vi "ADC_Monitor.vi"(0 "GPIB Address":T1=8, 5 "Chunk Size":i32=1000, 9 "Sample Rate (Hz)":dbl, 11 "error in (no error)":errorcluster, 12 "Local Client?":bool, 13 "Current Block No":i32) -> (6 "Barchart":cluster{i32, i32}(slide)={1, 0} scale=0.0..1048576.0, 15 "error out":errorcluster)   [LabVIEW 2010]
doc: "This VI starts a buffered analog input operation. This VI sets the scan rate and trigger conditions and then starts an acquisition.\n\nAI Start first checks to see if the input cluster error in indicates that an error has already occurred. If so, this VI does not start an acquisition, but passes the error information unmodified through error out. \n\nOtherwise, this VI calls several lower-level analog input VIs to start the buffered analog input acquisition. AI Start calls Analog Input Clock Config for the specified taskID to configure the acquisition to use the specified scan clock source (internal by default) and the specified scan rate.\n\nAI Start then calls Analog Input Trigger Config to set a trigger according to trigger type. If trigger type is 0, then it clears the trigger; otherwise it sets the specified type of trigger.\n\nFinally, AI Start calls Analog Input Control to start the acquisition, using total scans, pretrigger scans, and number of buffers to acquire to determine how much data to acquire.\n\nInput Values:\n\n(u32) taskID in: identifies the group and I/O operation.\n\n(i32) number of scans to aquire: the total number of scans to acquire before the acquisition is complete. The default input -1which tells LabVIEW to acquire exactly one buffer of data. The buffer size is specified when AI Config is called. The number of total scans includes any pretrigger scans requested. If you set number of scans to acquire to 0, LabVIEW acquires data indefinitely into the first (or only) buffer until you clear the acquisition with AI Clear. In this case, the VI ignores the pretrigger scans input.\n\n(sgl) scan rate: the number of scans per second to acquire. The default input is 1,000 scans/sec. Refer to the description of the Analog Input Clock Config VI for more options with alternate clock sources.\n\n(i32) number of buffers to acquire: needs to be changed only when you allocate more than one buffer with AI Config or Analog Input Buffer Config for multi-buffered acquisition (see Chapter 1 for a description of different types of I/O operation). If number of buffers to acquire is 0, LabVIEW acquires buffers of data indefinitely. Otherwise, LabVIEW acquires only the specified number of buffers. The default input is 1.\n\n(u16) scan clock source:\n 0: Do not change the clock source setting (default input). \n 1: Internal (default setting). \n 2: I/O connector. \n 3: RTSI connection. \n\n(u16) trigger type: \n 0: Do not change the trigger type setting (default input). \n 1: Analog trigger (default setting). \n 2: Digital trigger A. \n 3: Digital trigger A & B. \n 4: Scan clock gating. \n\n(i32) pretrigger scans: the number of scans to save in the buffer before the trigger. The default input is 0, which tells LabVIEW to acquire all data after the trigger.\n\n(u16) edge or slope:\n 0: Do not change the default setting (default input). \n 1: Rising edge for digital trigger or\n rising slope for analog trigger. \n 2: Falling edge for digital trigger or\n falling slope for analog trigger. \n\n(cluster) analog chan and level: a cluster of the following parameters that are used only when the trigger type is analog:\n\n (string) analog chan: specifies the analog channel\n that is the source of the trigger. Uses the same\n syntax described in the Analog Input Group Config VI,\n with the following exceptions. \n a) An empty string tells LabVIEW not to change \n the trigger source setting (default input).\n b) EXTx denotes an external analog input \n trigger, where x is the channel number.\n Currently, x must be 0. You can substitute\n the string EXTERNAL for EXT.\n \n (sgl) level: the scaled data value the analog source\n must cross for a trigger to occur. You must also\n specify whether level must be crossed on a rising \n or falling slope with the edge or slope input.\n The default input for level is 0.0.\n\n(cluster) additional trig params: a cluster of the following parameters: \n \n (sgl) hysteresis is expressed in scaled data values.\n The default input and setting are 0.0 V. \n \n (u16) coupling:\n 0: Do not change (default input). \n 1: DC. \n 2: AC. \n \n (sgl) delay: expressed in seconds.\n The default input and setting are 0.0 sec (no delay). \n \n (i32) skip count: the number of triggers to\n ignore before triggering the acquisition.\n The default input is -1, use the current default \n setting. The default setting is 0, don't skip \n any triggers. \n \n (sgl) time limit: time limit for software \n triggering. The default input is -1.0, use \n default setting. The default setting is 1.0Êsec. \n\n(cluster) error in: a cluster describing any error conditions prior to this VI's execution. The default input of this cluster is no error. If an error has already occurred, this VI does not start the acquisition, it just passes the values of taskID in and error in to taskID out and error out. The error in cluster contains the following parameters: \n\n (bool) status: TRUE if an error has occurred.\n If status is TRUE, this VI does not start the\n acquisition.\n\n (i32) code: the error code associated with an error.\n A value of 0 means no error, a negative value is an error,\n and a positive value is a warning.\n\n (string) source: an indication of where an \n error occurred, usually the name of the VI.\n\nOutput Values:\n\n(u32) taskID out: the same as taskID in; identifies the group and I/O operation.\n\n(sgl) actual scan rate: may differ slightly from the requested scan rate, depending on the hardware capabilities.\n\n(cluster) actual trigger params: may differ slightly from the requested trigger inputs, depending on the hardware capabilities. It contains the following parameters:\n \n (sgl) actual level: the analog trigger level used.\n \n (sgl) actual hysteresis: the hysteresis used. \n \n (sgl) actual delay: the trigger delay used. \n\n(cluster) error out: a cluster containing error information. If error in indicated an error, error out contains the same error information. Otherwise, it describes the error status of this VI. Use the General Error Handler utility VI to check the error at the end of your diagram. The error out cluster contains the following parameters: \n\n (bool) status: TRUE if an error has occurred.\n\n (i32) code: the error code associated with an error.\n A value of 0 means no error, a negative value is an error,\n and a positive value is a warning.\n\n (string) source: an indication of where an \n error occurred, usually the name of the VI."
uses:
  ADC_GPIB_address.ctl
panel:
  out "Unread samples":i32
  in  "stop":bool
  out "message":string
  # "Read marker"
  # "Write marker"
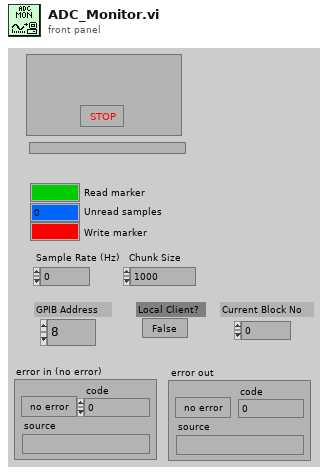
[diagram p1: front panel]
types:
  T1 = typedef "ADC_GPIB_address.ctl" = u8
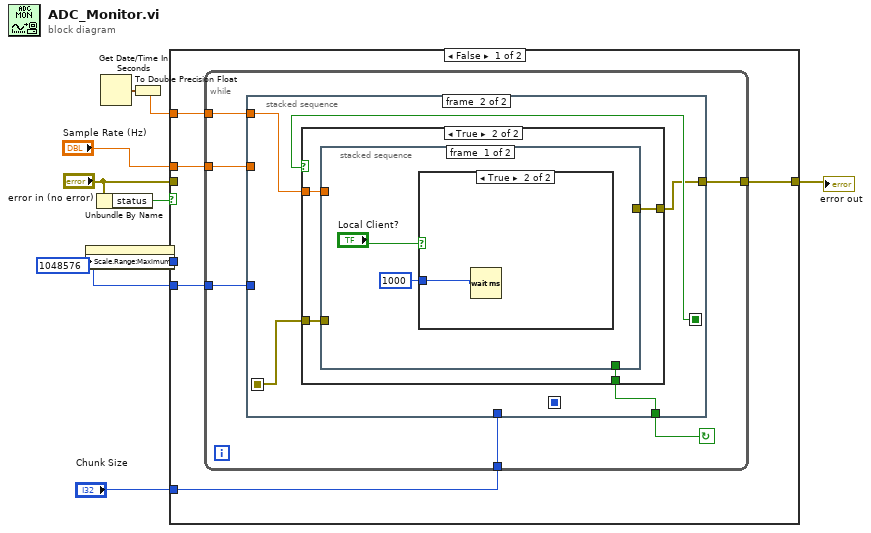
[diagram p0: block diagram]
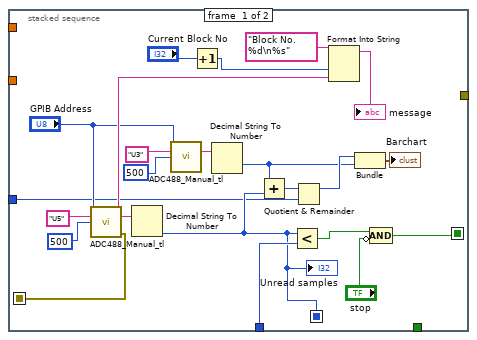
[diagram p2: hidden frame]
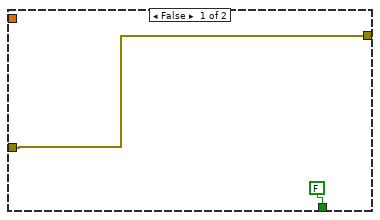
[diagram p3: hidden frame]
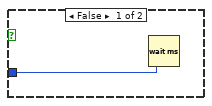
[diagram p4: hidden frame]
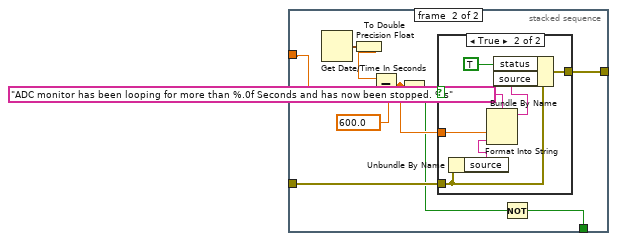
[diagram p5: hidden frame]
diagram:
  w3 = 1048576 ("y")
  n1 = property on="Barchart" class="Slide (strict)"("Scale.Range:Maximum"=w3) -> ()  [unwired: 2 in, 2 out]
  n2 = Unbundle By Name("error in (no error)") -> ("status"=w6:bool)
  n3 = Get Date/Time In Seconds() -> (seconds since 1Jan1904=w1:timestamp)
  n4 = To Double Precision Float(number=w1) -> (double precision float=w2:dbl)
  n5 = case shown="False" w6 {
    tunnel: [w10 w75] -> w8
    tunnel: "error in (no error)" -> [_ w75]
    tunnel: "Chunk Size" -> [w12 _]
    tunnel: w3 -> [_ _]
    tunnel: "Sample Rate (Hz)" -> [w13 _]
    tunnel: w3 -> [w11 _]
    tunnel: w2 -> [w9 _]
    frame False {
      n6 = while {
        tunnel: w11 -> [w16]
        tunnel: w13 -> [w17]
        tunnel: w12 -> [w19]
        tunnel: [w15] -> w10
        tunnel: w9 -> [w14]
        stop <- w18 continue-if-true
        n7 = stacked-sequence {
          seq-local: [w38 _] -> [_ w46]
          seq-local: [w25 _] -> [_ _]
          seq-local: [w20 _] -> [_ w45]
          tunnel: w19 -> [w41 _]
          tunnel: [_ w43] -> w18
          tunnel: w17 -> [_ _]
          tunnel: w16 -> [w23 _]
          tunnel: [_ w44] -> w15
          tunnel: w14 -> [_ w47]
          frame #0 {
            n8 = call "ADC488_Manual_tl.vi"("GPIB Address"="GPIB Address", "Command String"="U5", "Byte Count Requested"=500) -> ("Status String"=w32:string, "Response String"=w39:string, "error out"=w20:errorcluster)  [unwired: 4 in, 6 out]
            n9 = Decimal String To Number(string=w39) -> (number=w25:i32)  [unwired: 3 out]
            "Unread samples" <- w25
            n10 = call "ADC488_Manual_tl.vi"("GPIB Address"="GPIB Address", "Command String"="U3", "Byte Count Requested"=500) -> ("Response String"=w30:string)  [unwired: 4 in, 8 out]
            n11 = Increment(x="Current Block No") -> (x+1=w33:i32)
            n12 = Decimal String To Number(string=w30) -> (number=w21:i32)  [unwired: 3 out]
            n13 = Add(x=w21, y=w25) -> (x+y=w24:i32)
            n14 = Less?(x=w25, y=w41) -> (x < y?=w31:bool)
            n15 = Quotient & Remainder(x=w24, y=w23) -> (x-y*floor(x/y)=w22:i32)  [unwired: 1 out]
            n16 = Format Into String(format string="Block No. %d\n%s" ("Format String"), w33, w32) -> (resulting string=→"message":string)  [unwired: 2 in, 1 out]
            n17 = Bundle(w22, w21) -> (→"Barchart":cluster{i32, i32})  [unwired: 1 out]
            n18 = Compound Arithmetic op=AND(w31, invert "stop") -> (w38:bool)
          }
          frame #1 {
            n19 = case shown="True" w46 {
              tunnel: w47 -> [_ w53]
              tunnel: w45 -> [w48 w52]
              tunnel: [w48 w51] -> w44
              tunnel: [FALSE w50] -> w43
              frame False {
              }
              frame True {
                n20 = stacked-sequence {
                  tunnel: w53 -> [_ w65]
                  tunnel: w52 -> [_ w63]
                  tunnel: [_ w61] -> w51
                  tunnel: [_ w59] -> w50
                  frame #0 {
                    n21 = case shown="True" "Local Client?" {
                      tunnel: u32 1000 -> [w56 w57]
                      frame False {
                        n22 = Wait (ms)(milliseconds to wait=w56) -> ()  [unwired: 1 out]
                      }
                      frame True {
                        n23 = Wait (ms)(milliseconds to wait=w57) -> ()  [unwired: 1 out]
                      }
                    }
                  }
                  frame #1 {
                    n24 = Get Date/Time In Seconds() -> (seconds since 1Jan1904=w58:timestamp)
                    n25 = To Double Precision Float(number=w58) -> (double precision float=w66:dbl)
                    n26 = Subtract(x=w66, y=w65) -> (x-y=w62:dbl)
                    n27 = Greater?(x=w62, y=600.0) -> (0:w60:bool)
                    n28 = case shown="True" w60 {
                      tunnel: w63 -> [w67 w73]
                      tunnel: w62 -> [_ w72]
                      tunnel: [w67 w69] -> w61
                      frame False {
                      }
                      frame True {
                        n29 = Unbundle By Name(w73) -> ("source"=w70:string)
                        n30 = Format Into String(format string="ADC monitor has been looping for more than %.0f Seconds and has now been stopped. %s", w72, w70) -> (resulting string=w68:string)  [unwired: 2 in, 1 out]
                        n31 = Bundle By Name(cluster=w73, "status"=TRUE, "source"=w68) -> (w69:errorcluster)
                      }
                    }
                    n32 = Not(x=w60) -> (.not. x?=w59:bool)
                  }
                }
              }
            }
          }
        }
      }
    }
    frame True {
    }
  }
  "error out" <- w8
